vi "Audio.Test.vi"() -> ()   [LabVIEW 2018]
uses:
  <vilib>/sound2/lvsound2.llb/Sound Data Format.ctl
  <vilib>/sound2/lvsound2.llb/Sampling Mode.ctl
  <vilib>/Analysis/5stat.llb/RMS (DBL).vi
  <vilib>/sound2/lvsound2.llb/Sound Input Read (DBL).vi
  <vilib>/measure/maspectr.llb/FFT Spectrum (Mag-Phase) for 1 Chan.vi
  <vilib>/KATE/Time/Time Utils.lvlib
  <vilib>/Analysis/NI_AALPro.lvlib
  <vilib>/measure/NI_MAPro.lvlib
panel:
  in  "Limits":T1(array[cluster])=[{"FreqStart"=0.0, "FreqEnd"=1000.0, "Lim_dB"=-45.0, "Result"=TRUE}, {"FreqStart"=1000.0, "FreqEnd"=8000.0, "Lim_dB"=-60.0, "Result"=TRUE}] {"Lim_dB" format="%#.3f"; "FreqEnd" format="%#.3f"; "FreqStart" format="%#.3f"}
  out "FFT":cluster{"f0":dbl, "df":dbl, "magnitude":dbl[]}(graph)
  out "RMS":dbl format="%0.4f"
  out "Duration(s)":dbl format="%.2f"
  out "error out":errorcluster
  in  "stop":bool
  out "Amplitude":waveform(dbl)[](graph)
  in  "sound format":T2={"sample rate (S/s)"=22050.0, "number of channels"=2, "bits per sample"=16}
  # "Start(Hz)         End(Hz)         Limit (Max dB)"
  # "P/F"
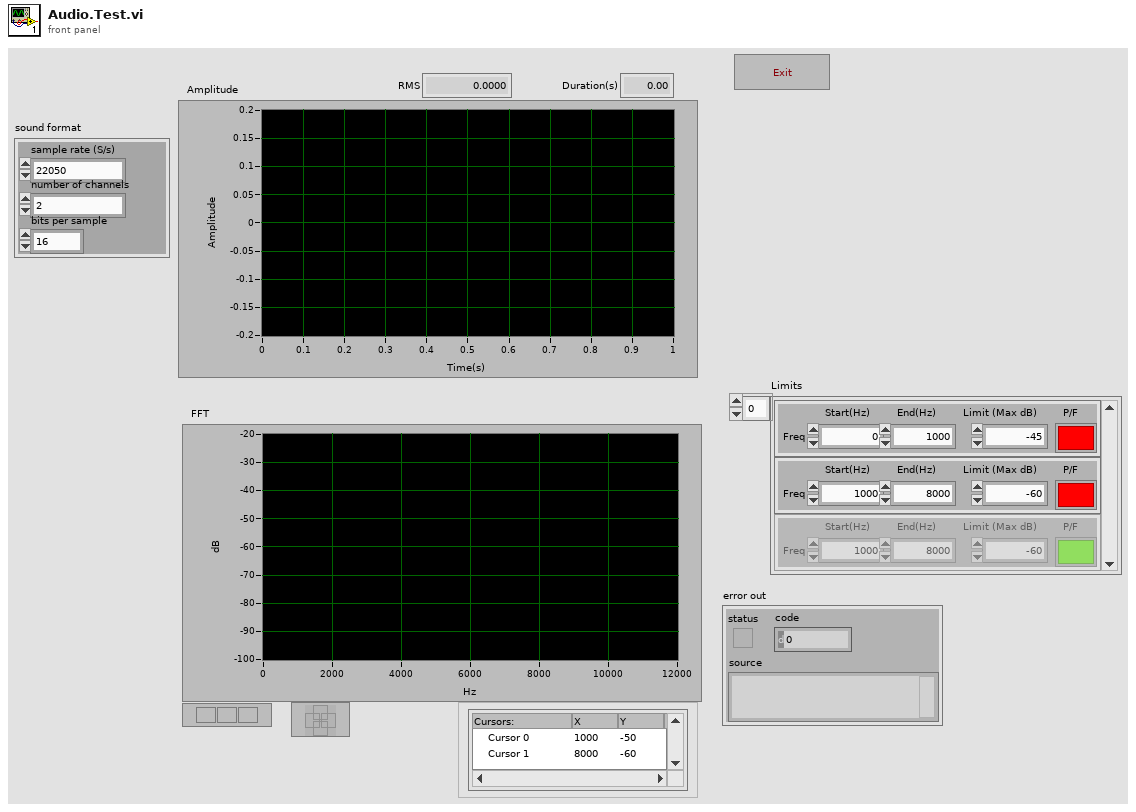
[diagram p1: front panel]
types:
  T1 = cluster{"FreqStart":dbl, "FreqEnd":dbl, "Lim_dB":dbl, "Result":bool}[]
  T2 = typedef "Sound Data Format.ctl" = cluster{"sample rate (S/s)":dbl, "number of channels":i32, "bits per sample":i32}
  T3 = typedef "Sampling Mode.ctl" = i32
  T4 = typedef "Sound Input Task ID.ctl" = u32
  T5 = cluster{"dB On (F)":bool, "unwrap phase (F)":bool, "convert to degree (F)":bool}
  T6 = cluster{"FreqStart":dbl, "FreqEnd":dbl, "Lim_dB":dbl, "Result":bool}
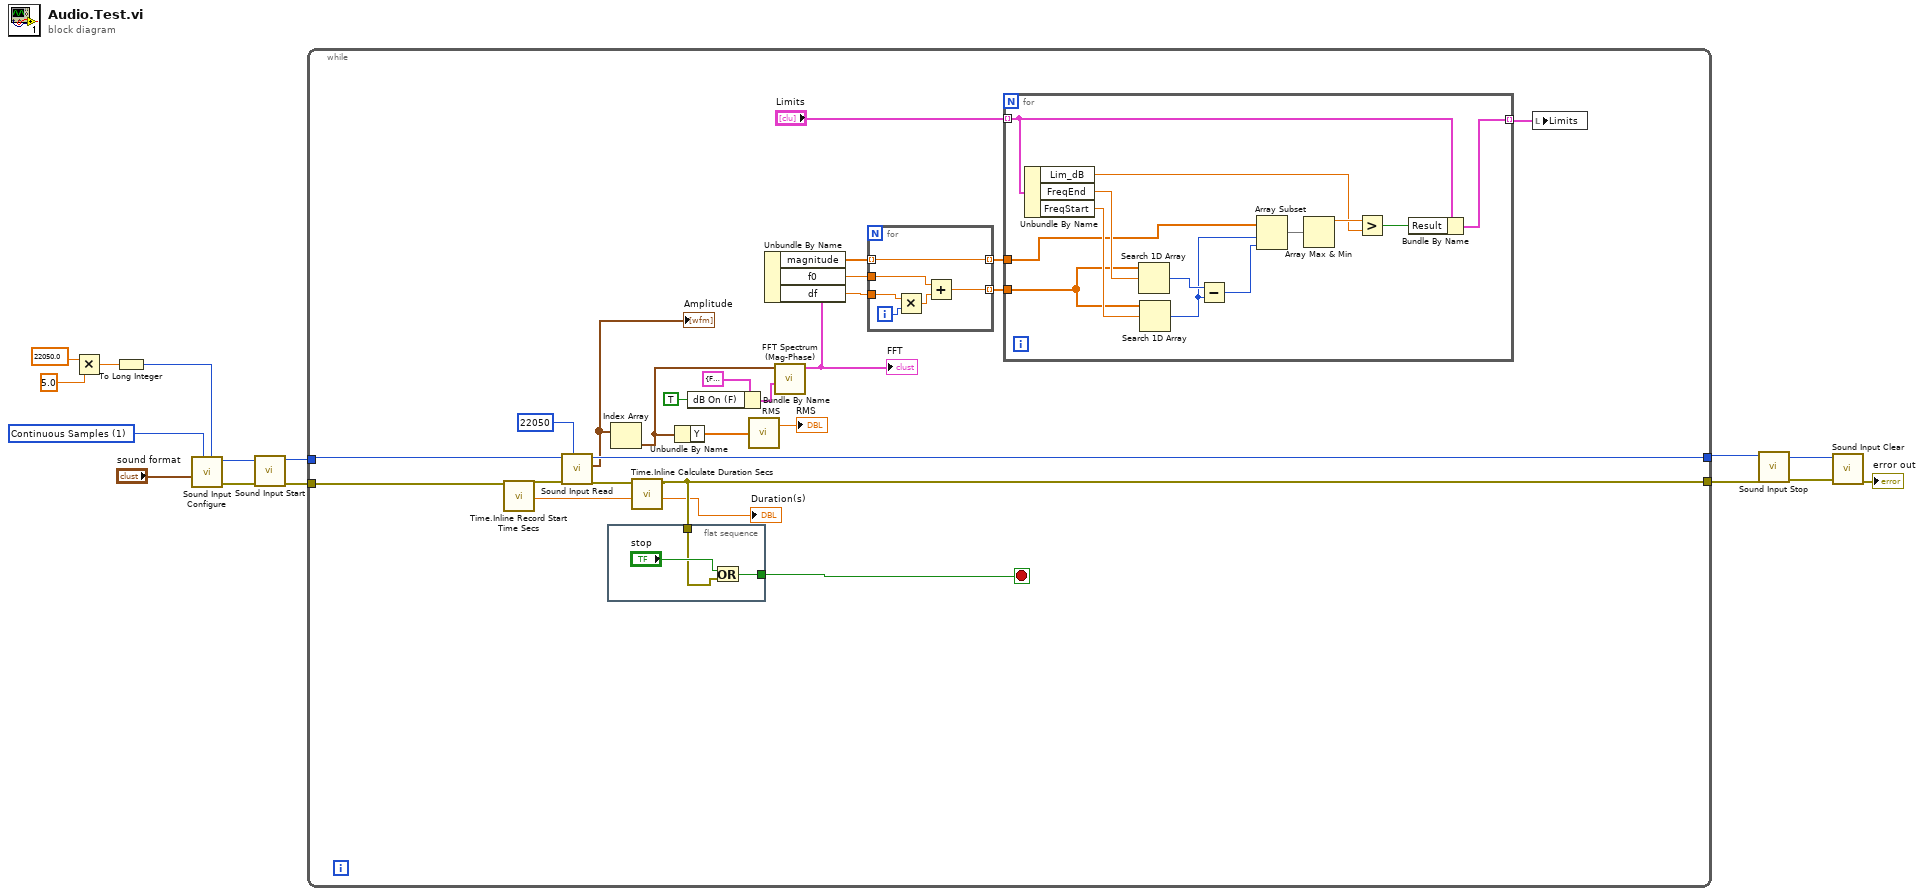
[diagram p0: block diagram]
diagram:
  w14 = T3 1 items=["Finite Samples", "Continuous Samples"] ("sample mode")
  n1 = Multiply(x=22050.0 ("sample rate (S/s)"), y=5.0) -> (x*y=w2:dbl)
  n2 = To Long Integer(number=w2) -> (32bit integer=w1:i32)
  n3 = call <vilib>:"Sound Input Configure.vi"("number of samples/ch"=w1, "sample mode"=w14, "sound format"="sound format") -> ("error out"=w12:errorcluster, "task ID"=w13:T4)  [unwired: 7 in]
  n4 = call <vilib>:"Sound Input Start.vi"("error in (no error)"=w12, "task ID"=w13) -> ("error out"=w10:errorcluster, "task ID out"=w11:T4)  [unwired: 8 in]
  n5 = while {
    tunnel: w11 -> [w40]
    tunnel: w10 -> [w37]
    tunnel: [w39] -> w9
    tunnel: [w34] -> w8
    stop <- w38 stop-if-true
    n6 = call <vilib>:"Time.Inline Record Start Time Secs.vi"("Error In Upper"=w37) -> ("Start(s)"=w33:dbl, "Error Out Upper"=w36:errorcluster)  [unwired: 8 in, 1 out]
    n7 = call-poly <vilib>:"Sound Input Read.vi"("number of samples/ch"=22050 ("sample rate (S/s)"), "error in (no error)"=w36, "task ID"=w40) -> ("error out"=w35:errorcluster, "data"=w29:waveform(dbl)[], "task ID out"=w39:T4)  [unwired: 6 in]
    "Amplitude" <- w29
    n8 = flat-sequence {
      tunnel: [w61] -> w38
      tunnel: w34 -> [w60]
      frame #0 {
        n9 = Or(x="stop", y=w60) -> (x .or. y?=w61:bool)
      }
    }
    n10 = Index Array(array=w29) -> (element=w28:waveform(dbl))  [unwired: 1 in]
    n11 = call <vilib>:"Time.Inline Calculate Duration Secs.vi"("Start(Sec)"=w33, "Error In Top"=w35) -> ("Duration(s)"=→"Duration(s)":dbl, "Error Out Top"=w34:errorcluster)  [unwired: 7 in, 1 out]
    n12 = Unbundle By Name(w28) -> ("Y"=w30:dbl[])
    n13 = Bundle By Name(cluster=T5 {"dB On (F)"=FALSE, "unwrap phase (F)"=FALSE, "convert to degree (F)"=FALSE} ("view"), "dB On (F)"=TRUE) -> (w26:T5)
    n14 = call-poly <vilib>:"RMS.vi"("X"=w30) -> ("rms value"=→"RMS":dbl)  [unwired: 1 out]
    n15 = call-poly <vilib>:"FFT Spectrum (Mag-Phase).vi"("view"=w26, "time signal"=w28) -> ("magnitude"=w22:cluster{"f0":dbl, "df":dbl, "magnitude":dbl[]})  [unwired: 5 in, 4 out]
    "FFT" <- w22
    n16 = Unbundle By Name(w22) -> ("magnitude"=w21:dbl[], "f0"=w20:dbl, "df"=w19:dbl)
    n17 = for {
      tunnel: w21 -> [w41] mode=indexing
      tunnel: w20 -> [w43]
      tunnel: w19 -> [w45]
      tunnel: [w42] -> w17 mode=indexing
      tunnel: [w41] -> w18 mode=indexing
      i -> [w46]
      n18 = Multiply(x=w45, y=w46) -> (x*y=w44:dbl)
      n19 = Add(x=w43, y=w44) -> (x+y=w42:dbl)
    }
    n20 = for {
      tunnel: "Limits" -> [w47] mode=indexing
      tunnel: w18 -> [w53]
      tunnel: w17 -> [w57]
      tunnel: [w49] -> w16 mode=indexing
      n21 = Unbundle By Name(w47) -> ("Lim_dB"=w50:dbl, "FreqEnd"=w59:dbl, "FreqStart"=w58:dbl)
      n22 = Search 1D Array(1D array=w57, element=w59) -> (index of element=w56:i32)  [unwired: 1 in]
      n23 = Search 1D Array(1D array=w57, element=w58) -> (index of element=w55:i32)  [unwired: 1 in]
      n24 = Subtract(x=w56, y=w55) -> (x-y=w54:i32)
      n25 = Array Subset(array=w53, index=w55, length=w54) -> (w52:dbl[])
      n26 = Array Max & Min(array=w52) -> (max value=w51:dbl)  [unwired: 3 out]
      n27 = Greater?(x=w51, y=w50) -> (0:w48:bool)
      n28 = Bundle By Name(cluster=w47, "Result"=w48) -> (w49:T6)
    }
    n29 = local write "Limits"(w16) -> ()
  }
  n30 = call <vilib>:"Sound Input Stop.vi"("error in (no error)"=w8, "task ID"=w9) -> ("error out"=w7:errorcluster, "task ID out"=w6:T4)  [unwired: 8 in]
  n31 = call <vilib>:"Sound Input Clear.vi"("error in (no error)"=w7, "task ID"=w6) -> ("error out"=→"error out":errorcluster)  [unwired: 9 in]
